vi "dfd_nMAC_DelayCounter.vi"(1 "reset":bool, 2 "data in":bool, 4 "#delay":fxp<+,16,16>) -> (7 "data out":bool)   [LabVIEW 2017]
uses:
  <vilib>/rvi/FXPMathLib/basic elements/FxpAddSub/XNode/nifxpmath_AddSub.xnode
  <vilib>/rvi/FXPMathLib/sim/FxpSim.dll
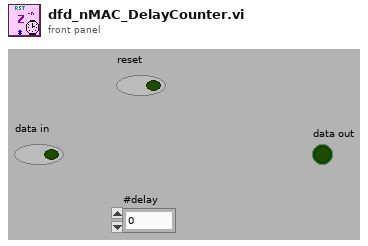
[diagram p1: front panel]
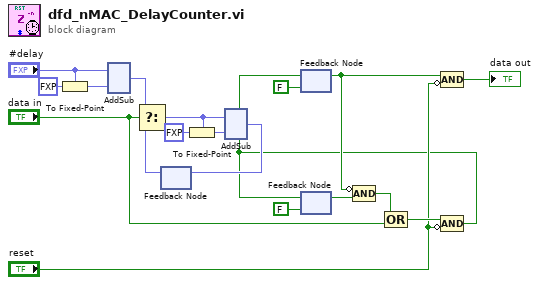
[diagram p0: block diagram]
diagram:
  n1 = To Fixed-Point(fixed-point type="#delay", number=fxp<+,1,1> 1.0 ("y")) -> (fixed-point=w4:fxp<+,16,16>)
  n2 = xnode "AddSub"("x"="#delay", "y"=w4) -> ("s"=w5:fxp<+,16,16>)  [unwired: 1 out]
  n3 = feedback #1() -> (w18:fxp<+,16,16>)  [unwired: 1 out]
  n4 = Select(t=w5, s="data in", f=w18) -> (s? t:f=w1:fxp<+,16,16>)
  n5 = To Fixed-Point(fixed-point type=w1, number=fxp<+,1,1> 0.0 ("y")) -> (fixed-point=w2:fxp<+,16,16>)
  n6 = feedback #2(FALSE ("borrow-out")) -> (w11:bool)
  n7 = feedback #3(FALSE ("borrow-out")) -> (w12:bool)
  n8 = Compound Arithmetic op=AND(invert w11, w12) -> (w10:bool)
  n9 = Compound Arithmetic op=OR(w10, "data in") -> (w9:bool)
  n10 = Compound Arithmetic op=AND(w11, invert "reset") -> (→"data out":bool)
  n11 = Compound Arithmetic op=AND(w9, invert "reset") -> (w7:bool)
  n12 = xnode "AddSub"("x"=w1, "y"=w2, "borrow-in"=w7) -> ("s"=w19:fxp<+,16,16>, "borrow-out"=w14:bool)
  n13 = feedback-in #1(w19) -> ()
  n14 = feedback-in #2(w14) -> ()
  n15 = feedback-in #3(w7) -> ()
